vi "Set Aircraft Info System Status.vi"(8 "Error In":errorcluster, 10 "System Status":string, 11 "Aircraft ID":u8) -> (0 "Error Out":errorcluster)   [LabVIEW 2014]
uses:
  Get Aircraft Information.vi
  Set Aircraft Information.vi
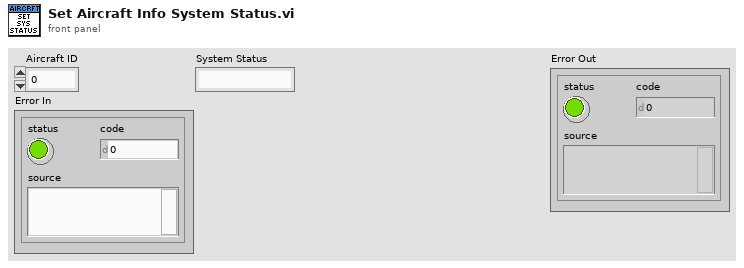
[diagram p1: front panel]
types:
  T1 = typedef "Drone Information.ctl" = cluster{"Heart Beat":bool, "Aircraft ID":u8, "Downlink Port":refnum<visa-resource-name>, "Tag ID":string, "System Status":string, "Base Mode":T2, "Armed/Disarmed":bool, "Battery Voltage":dbl, "Control Mode":T3, "Initialisation":u8, "Heart Beat Status":bool, "Uplink Port":refnum<visa-resource-name>, "UDP connection ID":refnum<k16>, "Connection Type":T4, "Mode":string, "UDP IP Address":string, "Mission Uploaded":bool}
  T2 = typedef "Base Mode.ctl" = cluster{"Custom Mode":bool, "Test Enabled":bool, "Autonomous Mode":bool, "Guided Mode":bool, "Stabilization Enabled":bool, "HIL Enabled":bool, "Manual Mode":bool, "Arm":bool}
  T3 = typedef "Aircraft Mode.ctl" = enum16{"Loiter", "Stabalise", "Failsafe", "Emergency Stop"}
  T4 = typedef "Telemetry Connection Type.ctl" = enum16{"Serial", "UDP", "TCP"}
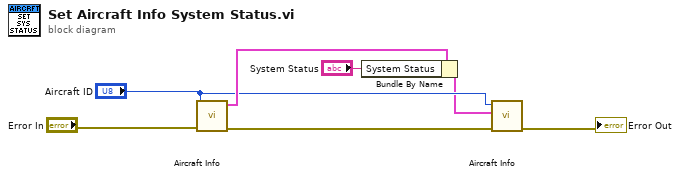
[diagram p0: block diagram]
diagram:
  n1 = call-poly "Aircraft Info.vi"("Error In"="Error In", "Aircraft ID"="Aircraft ID") -> ("Error Out"=w4:errorcluster, "Aircraft Information Out"=w6:T1)  [unwired: 8 in]
  n2 = Bundle By Name(cluster=w6, "System Status"="System Status") -> (w2:T1)
  n3 = call-poly "Aircraft Info.vi"("Error In"=w4, "Aircraft Information In"=w2, "Aircraft ID"="Aircraft ID") -> ("Error Out"=→"Error Out":errorcluster)  [unwired: 8 in]
